vi "3.1.vi"(0 "输入":dbl) -> (1 "正弦输出":dbl, 2 "余弦输出":dbl)   [LabVIEW 2017]
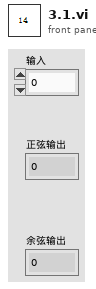
[diagram p1: front panel]
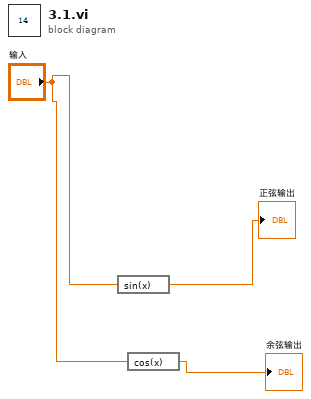
[diagram p0: block diagram]
diagram:
  n1 = expression code="sin(x)"("输入") -> (→"正弦输出":dbl)
  n2 = expression code="cos(x)"("输入") -> (→"余弦输出":dbl)
